vi "Get ni_measurementlink_measurement_v2_MeasureResponse.vi"(8 "error in (no error)":errorcluster, 11 "gRPCid":T1) -> (0 "error out":errorcluster, 2 "package_templatemessage":T2, 3 "gRPCid out":T4)   [LabVIEW 2020, in "MeasurementLink Measurement Service Base V2.lvlib"]
uses:
  MeasurementLink Measurement Service Base V2.lvlib
  <vilib>/gRPC/gRPC Server and Client Template [2]/grpcId.ctl
  ni_measurementlink_measurement_v2_MeasureResponse.ctl
  google_protobuf_Any.ctl
  <vilib>/gRPC/LabVIEW gRPC Library/Shared/grpcId.ctl
  ni_measurementlink_measurement_v2_MeasureResponse_Flat.ctl
  google_protobuf_Any_Flat.ctl
  2ed25e12-861d-4677-8ead-ace2906b2041.vi
  <vilib>/gRPC/LabVIEW gRPC Library/Shared/TranslateGrpcError.vi
  FlatToRichgoogle_protobuf_Any.vi
  <vilib>/gRPC/LabVIEW gRPC Library/Server API/Server/Get Server DLL Path.vi
  <vilib>/Utility/error.llb/Error Cluster From Error Code.vi
  <vilib>/Utility/error.llb/Simple Error Handler.vi
  <vilib>/gRPC/gRPC Server and Client Template [2]/grpc-lvsupport.lvlib
  <vilib>/gRPC/LabVIEW gRPC Library/grpc-lvsupport-release.lvlib
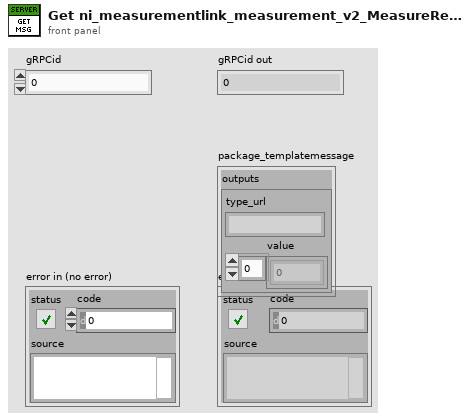
[diagram p1: front panel]
types:
  T1 = typedef "grpc-lvsupport-release.lvlib/grpcId.ctl" = u64
  T2 = typedef "MeasurementLink Measurement Service Base V2.lvlib/ni_measurementlink_measurement_v2_MeasureResponse.ctl" = cluster{"outputs":T3}
  T3 = typedef "MeasurementLink Measurement Service Base V2.lvlib/google_protobuf_Any.ctl" = cluster{"type_url":string, "value":u8[]}
  T4 = typedef "grpc-lvsupport.lvlib/grpcId.ctl" = u64
  T5 = typedef "MeasurementLink Measurement Service Base V2.lvlib/ni_measurementlink_measurement_v2_MeasureResponse_Flat.ctl" = cluster{"outputs":T6}
  T6 = typedef "MeasurementLink Measurement Service Base V2.lvlib/google_protobuf_Any_Flat.ctl" = cluster{"type_url":string, "value":u8[]}
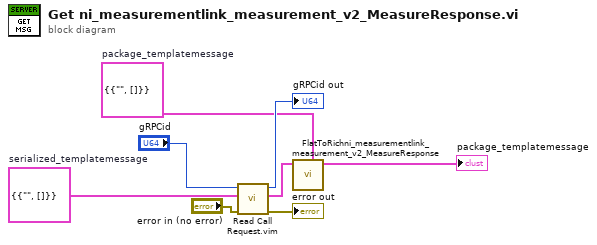
[diagram p0: block diagram]
diagram:
  w5 = T5 {"outputs"={"type_url"="", "value"=[]}}  # serialized_templatemessage
  w4 = T2 {"outputs"={"type_url"="", "value"=[]}}  # package_templatemessage
  n1 = call "Read Call Request.vim"("error in"="error in (no error)", "Request Type"=w5, "gRPCid in"="gRPCid") -> ("error out"=→"error out":errorcluster, "Request Data"=w3:T5, "gRPCid out"=→"gRPCid out":T1)  [unwired: 6 in]
  n2 = call "FlatToRichni_measurementlink_measurement_v2_MeasureResponse.vi"("OutputClusterType"=w4, "InputCluster"=w3) -> ("OutputCluster"=→"package_templatemessage":T2)  [unwired: 9 in]
